vi "Main_Sidestep_Prob.vi"() -> ()   [LabVIEW 2020]
panel:
  out "Num of Success":i16
  out "Prob_Success":dbl format="%#_3g"
  in  "Tab Control":T1(tab)
  out "XYグラフ":T2(graph)
  in  "Select Mol Posi":u16(ring)=4 items=["3 molecules", "5 molecules", "7 molecules", "9 molecules", "13 molecules", "17 molecules", ""]
  out "Particle State":T3(array[cluster])
  in  "SD":dbl=0.11000000000000001
  in  "Tau_On":i32=40
  in  "Tau_Off":i32=10
  in  "Sim Time":i32=55000
  in  "Asymmetry (X, Y)":dbl[](array[numeric])=[0.12000000000000001, 0.58]
  out "Count":i32
  in  "Torque 2":bool
  in  "Torque":dbl=-4.0
  in  "停止":bool
  in  "Rot_Noise for Cargo":bool
  in  "Width of Rot_Noise":dbl format="%#_13g"
  in  "Set_Roadblock(X, Y)":dbl[][](array[numeric])=[[30.0, -20.0], [50.0, 20.0]]
  in  "Iteration Sim":i32=300
  out "Counter":i32
  in  "Ini_Posi (3 mol)":dbl[][](array[numeric])=[[0.0, 0.0], [6.0, 0.0], [-6.0, 0.0]]
  in  "Ini_Posi (5 mol)":dbl[][](array[numeric])=[[0.0, 0.0], [6.0, 0.0], [-6.0, 0.0], [0.0, 6.0], [0.0, -6.0]]
  in  "Ini_Posi (9 mol)":dbl[][](array[numeric])=[[0.0, 0.0], [6.0, 0.0], [-6.0, 0.0], [0.0, 6.0], [0.0, -6.0], [6.0, 6.0], [6.0, -6.0], [-6.0, 6.0], [-6.0, -6.0]]
  in  "Ini_Posi (13 mol)":dbl[][](array[numeric])=[[0.0, 0.0], [6.0, 0.0], [-6.0, 0.0], [0.0, 6.0], [0.0, -6.0], [6.0, 6.0], [6.0, -6.0], [-6.0, 6.0], [-6.0, -6.0], [3.0, 3.0], [3.0, -3.0], [-3.0, 3.0], [-3.0, -3.0]]
  in  "Ini_Posi (13 mol#2)":dbl[][](array[numeric])=[[0.0, 0.0], [12.0, 3.0], [-12.0, 3.0], [12.0, -3.0], [-12.0, -3.0], [6.0, 0.0], [-6.0, 0.0], [0.0, -6.0], [0.0, 6.0], [6.0, 6.0], [6.0, -6.0], [-6.0, 6.0], [-6.0, -6.0], [3.0, 3.0], [3.0, -3.0], [-3.0, 3.0], [-3.0, -3.0]]
  in  "Ini_Posi (7 mol)":dbl[][](array[numeric])=[[0.0, 0.0], [5.0, 3.0], [-5.0, 3.0], [5.0, -3.0], [-5.0, -3.0], [0.0, 6.0], [0.0, -6.0]]
  out "Trajectory":cluster{"Position":dbl[], "Position":dbl[]}[](graph)
  out "Sidestep?":bool
  # "X_Bottom, Y_Left\n\nX_Top,  Y_Right"
  # "X_Center > X_bottom of the obstract"
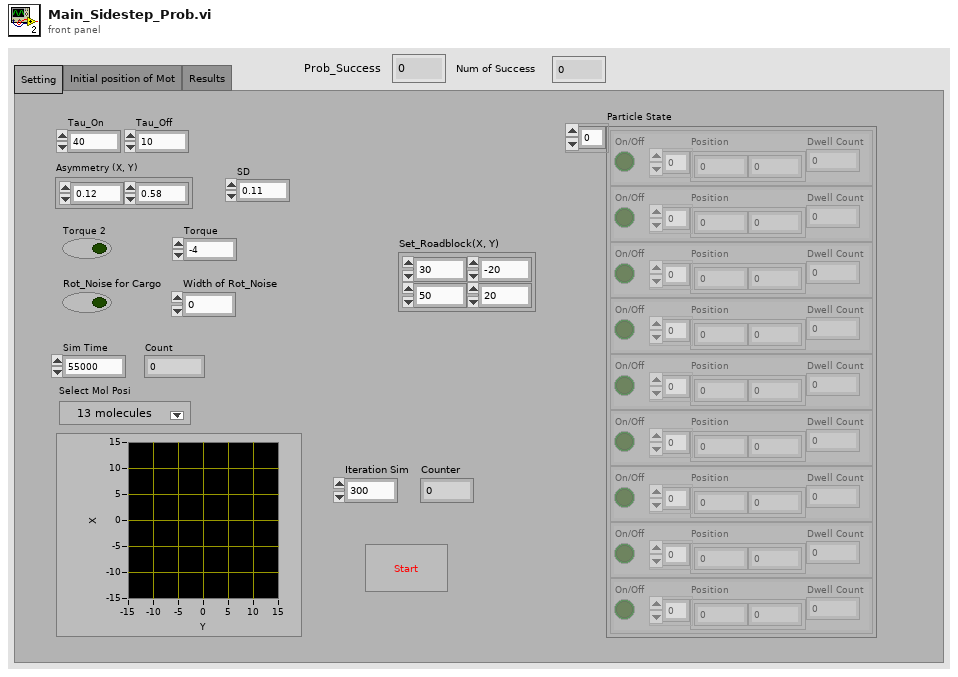
[diagram p1: front panel]
types:
  T1 = enum32{"Setting", "Initial position of Mot", "Results"}
  T2 = cluster{"Ini_Anchor_Posi (17 mol)":dbl[], "Ini_Anchor_Posi (17 mol)":dbl[]}
  T3 = cluster{"On/Off":bool, "Position":dbl[], "Dwell Count":i32}[]
  T4 = enum32{"Setting", "Initial position of Mot", "Results", "Results 2"}
  T5 = cluster{"Ini_Posi (13 mol#2)":dbl[], "Ini_Posi (13 mol#2)":dbl[]}
  T6 = cluster{"Center Position":dbl[], "Center Angle":dbl}
  T7 = cluster{"On/Off":bool, "Position":dbl[], "Next Dwell":i32}[]
  T8 = cluster{"On/Off":bool, "Position":dbl[], "Next Dwell":i32}
  T9 = cluster{"Posi_Roadblock":dbl[], "Posi_Roadblock":dbl[]}
  T10 = cluster{"Posi_Roadblock":dbl[], "Posi_Roadblock":dbl[]}[]
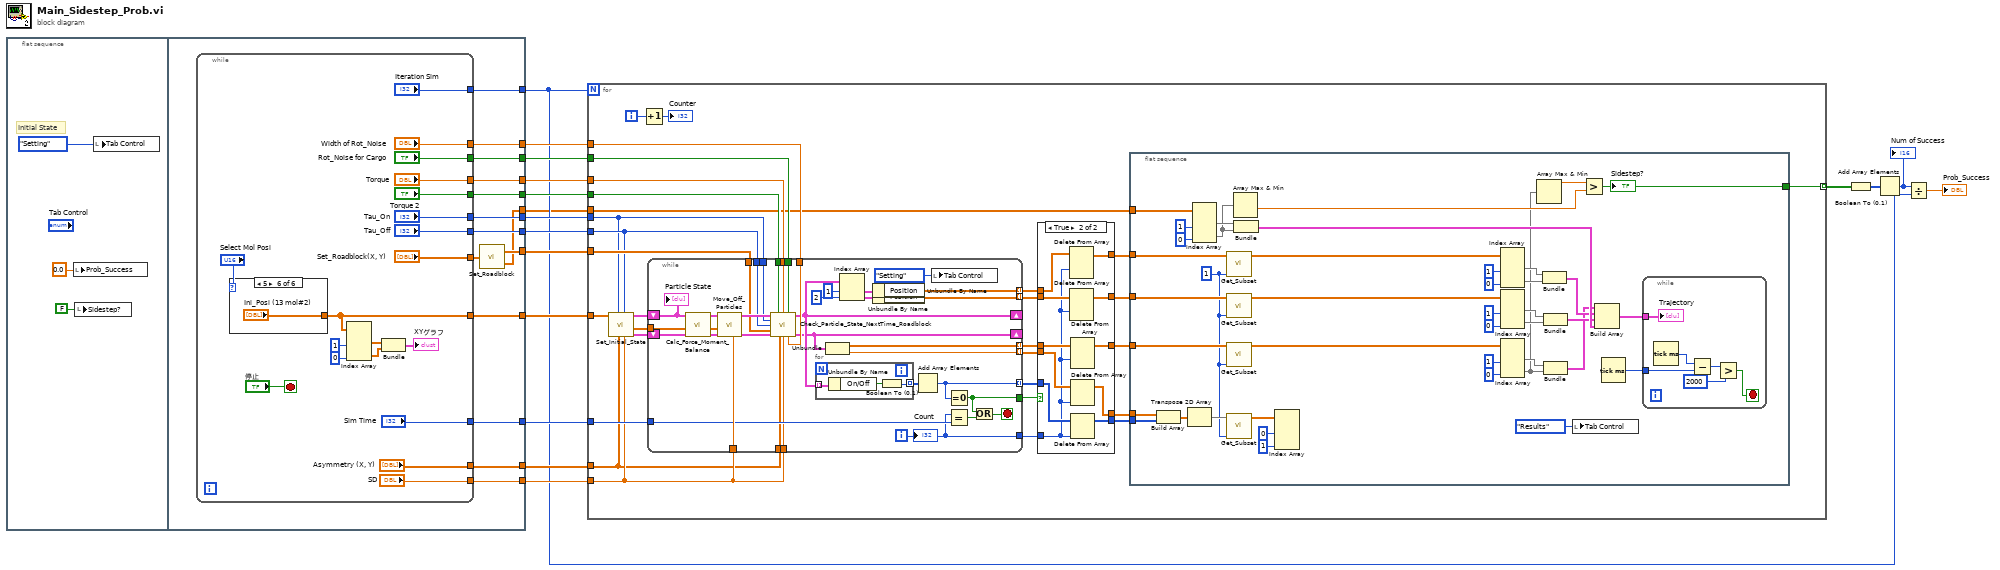
[diagram p0: block diagram]
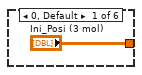
[diagram p3: hidden frame]
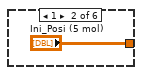
[diagram p4: hidden frame]
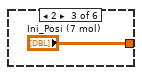
[diagram p5: hidden frame]
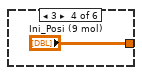
[diagram p6: hidden frame]
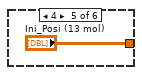
[diagram p7: hidden frame]
diagram:
  n1 = flat-sequence {
    tunnel: [w32] -> w11
    tunnel: [w34] -> w8
    tunnel: [w33] -> w10
    tunnel: [w31] -> w9
    tunnel: [w30] -> w17
    tunnel: [w29] -> w16
    tunnel: [w28] -> w15
    tunnel: [w27] -> w14
    tunnel: [w26] -> w13
    tunnel: [w22] -> w12
    tunnel: [w24] -> w7
    tunnel: [w23] -> w2
    tunnel: [w21] -> w1
    frame #0 {
      # "Initial State"
      n2 = local write "Prob_Success"(0.0 ("Prob_Success")) -> ()
      n3 = local write "Sidestep?"(FALSE ("Sidestep?")) -> ()
      n4 = local write "Tab Control"(T4."Setting" ("Tab Control")) -> ()
    }
    frame #1 {
      n5 = while {
        tunnel: ["Tau_On"] -> w34
        tunnel: ["Tau_Off"] -> w33
        tunnel: ["SD"] -> w32
        tunnel: ["Asymmetry (X, Y)"] -> w31
        tunnel: ["Torque 2"] -> w30
        tunnel: ["Torque"] -> w29
        tunnel: [w47] -> w24
        tunnel: ["Rot_Noise for Cargo"] -> w28
        tunnel: ["Width of Rot_Noise"] -> w27
        tunnel: ["Sim Time"] -> w26
        tunnel: ["Set_Roadblock(X, Y)"] -> w25
        tunnel: ["Iteration Sim"] -> w23
        stop <- "停止" stop-if-true
        n6 = case shown="5" "Select Mol Posi" {
          tunnel: ["Ini_Posi (3 mol)" "Ini_Posi (5 mol)" "Ini_Posi (7 mol)" "Ini_Posi (9 mol)" "Ini_Posi (13 mol)" "Ini_Posi (13 mol#2)"] -> w47
          frame 0, Default {
          }
          frame 1 {
          }
          frame 2 {
          }
          frame 3 {
          }
          frame 4 {
          }
          frame 5 {
          }
        }
        n7 = Index Array(array=w47, index (col) #1=1 ("無効な指標 (列)"), index (col) #2=0 ("指標 (列)")) -> (element #1=w42:dbl[], element #2=w41:dbl[])  [unwired: 2 in]
        n8 = Bundle("Ini_Posi (13 mol#2)"=w42, "Ini_Posi (13 mol#2)"=w41) -> (→"XYグラフ":T5)  [unwired: 1 in]
      }
      n9 = call "Set_Roadblock.vi"("Set_Obstacles(X, Y)"=w25) -> ("Posi_Roadblock_Bound"=w22:dbl[][], "Posi_Roadblock"=w21:dbl[][])
    }
  }
  n10 = for {
    N: w2 -> [_]
    tunnel: w17 -> [w89]
    tunnel: w16 -> [w88]
    tunnel: w15 -> [w76]
    tunnel: w14 -> [w75]
    tunnel: w13 -> [w74]
    tunnel: w12 -> [w72]
    tunnel: w11 -> [w71]
    tunnel: w10 -> [w70]
    tunnel: w9 -> [w69]
    tunnel: w8 -> [w68]
    tunnel: w7 -> [w67]
    tunnel: [w63] -> w6 mode=indexing
    tunnel: w1 -> [w60]
    i -> [w62]
    n11 = call "Set_Initial_State.vi"("SD"=w71, "Tau_Off"=w70, "Asymmetry (X, Y)"=w69, "Tau_On"=w68, "Ini_Anchor_Posi"=w67) -> ("Center State at T"=w66:T6, "Ini_Anchor_Posi"=w65:dbl[][], "On_Particle State"=w64:T3)  [unwired: 4 in]
    n12 = Increment(x=w62) -> (x+1=→"Counter":i32)
    n13 = while {
      tunnel: w65 -> [w140]
      shift-right: [w107] -> _
      shift-left: w66 -> [w138]
      shift-right: [w108] -> _
      shift-left: w64 -> [w139]
      tunnel: w71 -> [w132]
      tunnel: w68 -> [w115]
      tunnel: w70 -> [w114]
      tunnel: w69 -> [w111]
      tunnel: [w135] -> w86 mode=indexing
      tunnel: [w134] -> w85 mode=indexing
      tunnel: [w133] -> w84 mode=indexing
      tunnel: w71 -> [w110]
      tunnel: w89 -> [w119]
      tunnel: w88 -> [w118]
      tunnel: [w129] -> w83 mode=indexing
      tunnel: [w124] -> w82 mode=indexing
      tunnel: w74 -> [w125]
      tunnel: [w121] -> w87
      tunnel: [w120] -> w73
      tunnel: w76 -> [w117]
      tunnel: w75 -> [w109]
      tunnel: w72 -> [w112]
      i -> [w120]
      stop <- w122 stop-if-true
      n14 = call "Calc_Force_Moment_Balance.vi"("Center State at T"=w138, "Ini_Anchor_Posi"=w140, "On_Particle State"=w139) -> ("New Center State at T"=w130:T6, "Ini_Anchor_Posi"=w131:dbl[][], "On_Particle State"=w141:T3)  [unwired: 6 in]
      n15 = call "Move_Off_Particles.vi"("SD"=w132, "Center State at T"=w130, "Ini_Anchor_Posi"=w131, "Particle Posi at T"=w141) -> ("Center State at T"=w113:T6, "New Particle Posi at T"=w116:T7)  [unwired: 6 in]
      n16 = call "Check_Particle_State_NextTime_Roadblock.vi"("Particle State at T"=w116, "Torque?"=w119, "Torque"=w118, "Rot diffusion\nfor Cargo?"=w117, "Tau_On"=w115, "Tau_Off"=w114, "Posi_Obstacles"=w112, "Center State at T"=w113, "Asymmetry (X, Y)"=w111, "SD"=w110, "Rot diffusion\nfor Cargo"=w109) -> ("Particle State at T+1"=w108:T7, "New Center State at T"=w107:T6)  [unwired: 3 in]
      n17 = for {
        tunnel: w108 -> [w144] mode=indexing
        tunnel: [w142] -> w128 mode=indexing
        n18 = Unbundle By Name(w144) -> ("On/Off"=w143:bool)
        n19 = Boolean To (0,1)(Boolean=w143) -> (0, 1=w142:i16)
      }
      n20 = Unbundle(w107) -> ("Center Position"=w133:dbl[], "Center Angle"=w129:dbl)
      n21 = Index Array(array=w108, index #1=1 ("index"), index #2=2 ("index")) -> (element #1=w137:T8, element #2=w136:T8)
      n22 = Unbundle By Name(w137) -> ("Position"=w135:dbl[])
      n23 = Unbundle By Name(w136) -> ("Position"=w134:dbl[])
      n24 = Add Array Elements(numeric array=w128) -> (sum=w124:i16)
      n25 = local write "Tab Control"(T4."Setting" ("Tab Control")) -> ()
      n26 = Equal To 0?(x=w124) -> (x = 0?=w121:bool)
      n27 = Equal?(x=w120, y=w125) -> (x = y?=w123:bool)
      n28 = Or(x=w121, y=w123) -> (x .or. y?=w122:bool)
      "Particle State" <- w139
      "Count" <- w120
    }
    n29 = case shown="TRUE" w87 {
      tunnel: w86 -> [w94 w105]
      tunnel: w85 -> [w93 w104]
      tunnel: w73 -> [_ w100]
      tunnel: w84 -> [w92 w103]
      tunnel: w83 -> [w91 w102]
      tunnel: w82 -> [w90 w101]
      tunnel: [w90 w99] -> w81
      tunnel: [w91 w98] -> w80
      tunnel: [w92 w97] -> w79
      tunnel: [w93 w96] -> w78
      tunnel: [w94 w95] -> w77
      frame False {
      }
      frame True {
        n30 = Delete From Array(array=w105, index (row)=w100) -> (array with subset deleted=w95:dbl[][])  [unwired: 2 in, 1 out]
        n31 = Delete From Array(array=w104, index (row)=w100) -> (array with subset deleted=w96:dbl[][])  [unwired: 2 in, 1 out]
        n32 = Delete From Array(array=w103, index (row)=w100) -> (array with subset deleted=w97:dbl[][])  [unwired: 2 in, 1 out]
        n33 = Delete From Array(array=w102, index=w100) -> (array with subset deleted=w98:dbl[])  [unwired: 1 in, 1 out]
        n34 = Delete From Array(array=w101, index=w100) -> (array with subset deleted=w99:i16[])  [unwired: 1 in, 1 out]
      }
    }
    n35 = flat-sequence {
      tunnel: w77 -> [w171]
      tunnel: w78 -> [w185]
      tunnel: w79 -> [w184]
      tunnel: w80 -> [w183]
      tunnel: w81 -> [w177]
      tunnel: w60 -> [w170]
      tunnel: [w163] -> w63
      frame #0 {
        w172 = 1
        n36 = Build Array(w183, w177) -> (w182:dbl[][])
        n37 = Transpose 2D Array(2D array=w182) -> (transposed array=w181:dbl[][])
        n38 = Index Array(array=w170, index (col) #1=1 ("無効な指標 (列)"), index (col) #2=0 ("指標 (列)")) -> (element #1=w167:dbl[], element #2=w165:dbl[])  [unwired: 2 in]
        n39 = call "Get_Subset.vi"("index"=w172, "Input"=w171) -> ("Output"=w176:dbl[][])  [unwired: 9 in]
        n40 = call "Get_Subset.vi"("index"=w172, "Input"=w185) -> ("Output"=w175:dbl[][])  [unwired: 9 in]
        n41 = call "Get_Subset.vi"("index"=w172, "Input"=w184) -> ("Output"=w174:dbl[][])  [unwired: 9 in]
        n42 = call "Get_Subset.vi"("index"=w172, "Input"=w181) -> ("Output"=w180:dbl[][])  [unwired: 9 in]
        n43 = Array Max & Min(array=w165) -> (min value=w164:dbl)  [unwired: 3 out]
        n44 = Bundle("Posi_Roadblock"=w167, "Posi_Roadblock"=w165) -> (w166:T9)  [unwired: 1 in]
        n45 = Index Array(array=w180, index (col) #1=0 ("disabled index (col)"), index (col) #2=1 ("index (col)")) -> ()  [unwired: 2 in, 2 out]
        n46 = Index Array(array=w176, index (col) #1=1 ("disabled index (col)"), index (col) #2=0 ("index (col)")) -> (element #1=w150:dbl[], element #2=w158:dbl[])  [unwired: 2 in]
        n47 = Index Array(array=w175, index (col) #1=1 ("disabled index (col)"), index (col) #2=0 ("index (col)")) -> (element #1=w151:dbl[], element #2=w157:dbl[])  [unwired: 2 in]
        n48 = Index Array(array=w174, index (col) #1=1 ("disabled index (col)"), index (col) #2=0 ("index (col)")) -> (element #1=w148:dbl[], element #2=w147:dbl[])  [unwired: 2 in]
        n49 = Array Max & Min(array=w147) -> (max value=w146:dbl)  [unwired: 3 out]
        n50 = Bundle("Output"=w150, "Output"=w158) -> (w156:cluster{"Output":dbl[], "Output":dbl[]})  [unwired: 1 in]
        n51 = Bundle("Output"=w151, "Output"=w157) -> (w155:cluster{"Output":dbl[], "Output":dbl[]})  [unwired: 1 in]
        n52 = Bundle("Output"=w148, "Output"=w147) -> (w152:cluster{"Output":dbl[], "Output":dbl[]})  [unwired: 1 in]
        n53 = local write "Tab Control"(T4."Results" ("Tab Control")) -> ()
        n54 = Greater?(x=w146, y=w164) -> (0:w163:bool)
        "Sidestep?" <- w163
        n55 = Build Array(w152, w156, w155, w166) -> (w149:T10)
        n56 = Tick Count (ms)() -> (millisecond timer value=w145:u32)
        n57 = while {
          tunnel: w149 -> [w191]
          tunnel: w145 -> [w189]
          stop <- w186 stop-if-true
          n58 = Tick Count (ms)() -> (millisecond timer value=w190:u32)
          n59 = Subtract(x=w190, y=w189) -> (x-y=w188:u32)
          n60 = Greater?(x=w188, y=u32 2000) -> (0:w186:bool)
          "Trajectory" <- w191
        }
      }
    }
  }
  n61 = Boolean To (0,1)(Boolean=w6) -> (0, 1=w5:i16[])
  n62 = Add Array Elements(numeric array=w5) -> (sum=w4:i16)
  "Num of Success" <- w4
  n63 = Divide(x=w4, y=w2) -> (x/y=→"Prob_Success":dbl)
